vi "Lab Panel V5.29.vi"() -> ()   [LabVIEW 2013] (continued)
                            n2522 = Build Array(w4624) -> (w4612:dbl[])
                            n2523 = Build Array(w4625) -> (w4611:dbl[])
                            n2524 = Build Array(w4620) -> (w4616:dbl[])
                            n2525 = Build Array(w4618) -> (w4615:dbl[])
                            n2526 = Build Array(w4623) -> (w4610:dbl[])
                            n2527 = Build Array("AMPS ON", "AMPS OFF", "VOLTS", "PF", "TEMP Live", "TEMP Neut", "CYCLE") -> (w4593:string[])
                            n2528 = Bundle By Name("Y"=w4616, "t0"=w4609) -> (w4608:waveform(dbl))  [unwired: 1 in]
                            n2529 = Bundle By Name("Y"=w4615, "t0"=w4609) -> (w4607:waveform(dbl))  [unwired: 1 in]
                            n2530 = Bundle By Name("Y"=w4614, "t0"=w4609) -> (w4606:waveform(dbl))  [unwired: 1 in]
                            n2531 = Bundle By Name("Y"=w4613, "t0"=w4609) -> (w4605:waveform(dbl))  [unwired: 1 in]
                            n2532 = Bundle By Name("Y"=w4612, "t0"=w4609) -> (w4604:waveform(dbl))  [unwired: 1 in]
                            n2533 = Bundle By Name("Y"=w4611, "t0"=w4609) -> (w4603:waveform(dbl))  [unwired: 1 in]
                            n2534 = Bundle By Name("Y"=w4610, "t0"=w4609) -> (w4602:waveform(dbl))  [unwired: 1 in]
                            n2535 = Build Array(w4608, w4607, w4606, w4605, w4604, w4603, w4602) -> (w4601:waveform(dbl)[])
                            n2536 = TDMS Write(0:w4622, 5:"TEST VALUES", 7:w4593, 9:w4601) -> (4:w4592:refnum<k34>, 6:w4591:string, 15:w4590:errorcluster)  [unwired: 2 in, 1 out]
                            n2537 = TDMS Write(0:w4592, 5:w4591, 7:"TIME", 9:w4588, 11:w4590) -> (15:w4587:errorcluster)  [unwired: 1 in, 3 out]
                            n2538 = local write "data file error"(w4587) -> ()
                          }
                        }
                      }
                    }
                  }
                }
              }
              frame #8 {
                n2539 = case shown="True" w4626 {
                  tunnel: w4630 -> [_ w4635]
                  tunnel: w4629 -> [_ w4634]
                  tunnel: w4628 -> [_ w4632]
                  tunnel: w4627 -> [_ w4631]
                  frame False {
                  }
                  frame True {
                    n2540 = local read "DISP LAB05-1"() -> (w4636:T4)
                    n2541 = local read "SIG LAB05-1"() -> (w4637:T2)
                    n2542 = local read "ON L05-1"() -> (w4633:cluster{"amps":dbl, "volts":dbl, "pf":dbl})
                    n2543 = Unbundle(w4637) -> ("AMPS"=w4643:dbl, "VOLTS"=w4641:dbl, "PF"=w4640:dbl, "Tmp Live"=w4639:dbl, "Tmp Neut"=w4642:dbl)
                    n2544 = Unbundle(w4636) -> ("CYCLE"=w4638:dbl)  [unwired: 2 out]
                    n2545 = stacked-sequence {
                      tunnel: w4643 -> [w4647 w4666]
                      tunnel: w4642 -> [_ w4665]
                      tunnel: w4641 -> [w4646 w4664]
                      tunnel: w4640 -> [w4645 w4663]
                      tunnel: w4639 -> [_ w4662]
                      tunnel: w4638 -> [_ w4661]
                      tunnel: w4635 -> [_ w4660]
                      tunnel: w4634 -> [w4648 _]
                      tunnel: w4633 -> [w4644 w4658]
                      tunnel: w4632 -> [_ w4659]
                      tunnel: w4631 -> [_ w4654]
                      frame #0 {
                        n2546 = case shown="True" w4648 {
                          tunnel: w4647 -> [_ w4653]
                          tunnel: w4646 -> [_ w4652]
                          tunnel: w4645 -> [_ w4651]
                          tunnel: w4644 -> [_ w4649]
                          frame False {
                          }
                          frame True {
                            n2547 = Bundle(cluster=w4649, "amps"=w4653, "volts"=w4652, "pf"=w4651) -> (w4650:cluster{"amps":dbl, "volts":dbl, "pf":dbl})
                            n2548 = local write "ON L05-1"(w4650) -> ()
                          }
                        }
                      }
                      frame #1 {
                        n2549 = Unbundle(w4658) -> ("amps"=w4657:dbl, "volts"=w4656:dbl, "pf"=w4655:dbl)
                        n2550 = case shown="True" w4659 {
                          tunnel: w4666 -> [_ w4698]
                          tunnel: w4665 -> [_ w4705]
                          tunnel: w4664 -> [_ _]
                          tunnel: w4663 -> [_ _]
                          tunnel: w4662 -> [_ w4704]
                          tunnel: w4661 -> [_ w4703]
                          tunnel: w4660 -> [_ w4668]
                          tunnel: w4657 -> [_ w4700]
                          tunnel: w4656 -> [_ w4699]
                          tunnel: w4655 -> [_ w4697]
                          tunnel: w4654 -> [_ w4689]
                          frame False {
                          }
                          frame True {
                            n2551 = local read "TDMS LAB05-1"() -> (w4702:refnum<k34>)
                            n2552 = Build Array(w4699) -> (w4694:dbl[])
                            n2553 = Build Array(w4697) -> (w4693:dbl[])
                            n2554 = Build Array(w4704) -> (w4692:dbl[])
                            n2555 = Build Array(w4705) -> (w4691:dbl[])
                            n2556 = Build Array(w4700) -> (w4696:dbl[])
                            n2557 = Build Array(w4698) -> (w4695:dbl[])
                            n2558 = Build Array(w4703) -> (w4690:dbl[])
                            n2559 = Build Array("AMPS ON", "AMPS OFF", "VOLTS", "PF", "TEMP Live", "TEMP Neut", "CYCLE") -> (w4673:string[])
                            n2560 = Bundle By Name("Y"=w4696, "t0"=w4689) -> (w4688:waveform(dbl))  [unwired: 1 in]
                            n2561 = Bundle By Name("Y"=w4695, "t0"=w4689) -> (w4687:waveform(dbl))  [unwired: 1 in]
                            n2562 = Bundle By Name("Y"=w4694, "t0"=w4689) -> (w4686:waveform(dbl))  [unwired: 1 in]
                            n2563 = Bundle By Name("Y"=w4693, "t0"=w4689) -> (w4685:waveform(dbl))  [unwired: 1 in]
                            n2564 = Bundle By Name("Y"=w4692, "t0"=w4689) -> (w4684:waveform(dbl))  [unwired: 1 in]
                            n2565 = Bundle By Name("Y"=w4691, "t0"=w4689) -> (w4683:waveform(dbl))  [unwired: 1 in]
                            n2566 = Bundle By Name("Y"=w4690, "t0"=w4689) -> (w4682:waveform(dbl))  [unwired: 1 in]
                            n2567 = Build Array(w4688, w4687, w4686, w4685, w4684, w4683, w4682) -> (w4681:waveform(dbl)[])
                            n2568 = TDMS Write(0:w4702, 5:"TEST VALUES", 7:w4673, 9:w4681) -> (4:w4672:refnum<k34>, 6:w4671:string, 15:w4670:errorcluster)  [unwired: 2 in, 1 out]
                            n2569 = TDMS Write(0:w4672, 5:w4671, 7:"TIME", 9:w4668, 11:w4670) -> (15:w4667:errorcluster)  [unwired: 1 in, 3 out]
                            n2570 = local write "data file error"(w4667) -> ()
                          }
                        }
                      }
                    }
                  }
                }
              }
              frame #9 {
                n2571 = case shown="True" w4706 {
                  tunnel: w4710 -> [_ w4715]
                  tunnel: w4709 -> [_ w4714]
                  tunnel: w4708 -> [_ w4712]
                  tunnel: w4707 -> [_ w4711]
                  frame False {
                  }
                  frame True {
                    n2572 = local read "DISP LAB05-2"() -> (w4716:T4)
                    n2573 = local read "SIG LAB05-2"() -> (w4717:T2)
                    n2574 = local read "ON L05-2"() -> (w4713:cluster{"amps":dbl, "volts":dbl, "pf":dbl})
                    n2575 = Unbundle(w4717) -> ("AMPS"=w4723:dbl, "VOLTS"=w4721:dbl, "PF"=w4720:dbl, "Tmp Live"=w4719:dbl, "Tmp Neut"=w4722:dbl)
                    n2576 = Unbundle(w4716) -> ("CYCLE"=w4718:dbl)  [unwired: 2 out]
                    n2577 = stacked-sequence {
                      tunnel: w4723 -> [w4727 w4746]
                      tunnel: w4722 -> [_ w4745]
                      tunnel: w4721 -> [w4726 w4744]
                      tunnel: w4720 -> [w4725 w4743]
                      tunnel: w4719 -> [_ w4742]
                      tunnel: w4718 -> [_ w4741]
                      tunnel: w4715 -> [_ w4740]
                      tunnel: w4714 -> [w4728 _]
                      tunnel: w4713 -> [w4724 w4738]
                      tunnel: w4712 -> [_ w4739]
                      tunnel: w4711 -> [_ w4734]
                      frame #0 {
                        n2578 = case shown="True" w4728 {
                          tunnel: w4727 -> [_ w4733]
                          tunnel: w4726 -> [_ w4732]
                          tunnel: w4725 -> [_ w4731]
                          tunnel: w4724 -> [_ w4729]
                          frame False {
                          }
                          frame True {
                            n2579 = Bundle(cluster=w4729, "amps"=w4733, "volts"=w4732, "pf"=w4731) -> (w4730:cluster{"amps":dbl, "volts":dbl, "pf":dbl})
                            n2580 = local write "ON L05-2"(w4730) -> ()
                          }
                        }
                      }
                      frame #1 {
                        n2581 = Unbundle(w4738) -> ("amps"=w4737:dbl, "volts"=w4736:dbl, "pf"=w4735:dbl)
                        n2582 = case shown="True" w4739 {
                          tunnel: w4746 -> [_ w4778]
                          tunnel: w4745 -> [_ w4785]
                          tunnel: w4744 -> [_ _]
                          tunnel: w4743 -> [_ _]
                          tunnel: w4742 -> [_ w4784]
                          tunnel: w4741 -> [_ w4783]
                          tunnel: w4740 -> [_ w4748]
                          tunnel: w4737 -> [_ w4780]
                          tunnel: w4736 -> [_ w4779]
                          tunnel: w4735 -> [_ w4777]
                          tunnel: w4734 -> [_ w4769]
                          frame False {
                          }
                          frame True {
                            n2583 = local read "TDMS LAB05-2"() -> (w4782:refnum<k34>)
                            n2584 = Build Array(w4779) -> (w4774:dbl[])
                            n2585 = Build Array(w4777) -> (w4773:dbl[])
                            n2586 = Build Array(w4784) -> (w4772:dbl[])
                            n2587 = Build Array(w4785) -> (w4771:dbl[])
                            n2588 = Build Array(w4780) -> (w4776:dbl[])
                            n2589 = Build Array(w4778) -> (w4775:dbl[])
                            n2590 = Build Array(w4783) -> (w4770:dbl[])
                            n2591 = Build Array("AMPS ON", "AMPS OFF", "VOLTS", "PF", "TEMP Live", "TEMP Neut", "CYCLE") -> (w4753:string[])
                            n2592 = Bundle By Name("Y"=w4776, "t0"=w4769) -> (w4768:waveform(dbl))  [unwired: 1 in]
                            n2593 = Bundle By Name("Y"=w4775, "t0"=w4769) -> (w4767:waveform(dbl))  [unwired: 1 in]
                            n2594 = Bundle By Name("Y"=w4774, "t0"=w4769) -> (w4766:waveform(dbl))  [unwired: 1 in]
                            n2595 = Bundle By Name("Y"=w4773, "t0"=w4769) -> (w4765:waveform(dbl))  [unwired: 1 in]
                            n2596 = Bundle By Name("Y"=w4772, "t0"=w4769) -> (w4764:waveform(dbl))  [unwired: 1 in]
                            n2597 = Bundle By Name("Y"=w4771, "t0"=w4769) -> (w4763:waveform(dbl))  [unwired: 1 in]
                            n2598 = Bundle By Name("Y"=w4770, "t0"=w4769) -> (w4762:waveform(dbl))  [unwired: 1 in]
                            n2599 = Build Array(w4768, w4767, w4766, w4765, w4764, w4763, w4762) -> (w4761:waveform(dbl)[])
                            n2600 = TDMS Write(0:w4782, 5:"TEST VALUES", 7:w4753, 9:w4761) -> (4:w4752:refnum<k34>, 6:w4751:string, 15:w4750:errorcluster)  [unwired: 2 in, 1 out]
                            n2601 = TDMS Write(0:w4752, 5:w4751, 7:"TIME", 9:w4748, 11:w4750) -> (15:w4747:errorcluster)  [unwired: 1 in, 3 out]
                            n2602 = local write "data file error"(w4747) -> ()
                          }
                        }
                      }
                    }
                  }
                }
              }
            }
          }
          frame #15 {
            # "display test values on chart"
            n2603 = local read "jig cycle"() -> (w4790:dbl)
            n2604 = local read "on loops"() -> (w4792:dbl)
            n2605 = Add(x=w4792, y=4) -> (x+y=w4789:dbl)
            n2606 = Equal?(x=w4790, y=3) -> (x = y?=w4788:bool)
            n2607 = Equal?(x=w4790, y=w4789) -> (x = y?=w4787:bool)
            n2608 = Or(x=w4788, y=w4787) -> (x .or. y?=w4786:bool)
            "graph flag" <- w4786
            n2609 = global write "Global display 3.vi" "graph flag"(w4786) -> ()
            n2610 = case shown="True" w4786 {
              frame False {
              }
              frame True {
                n2611 = local read "SIG LAB05-1"() -> (w4835:T2)
                n2612 = local read "SIG LAB04-2"() -> (w4836:T2)
                n2613 = local read "SIG LAB05-2"() -> (w4834:T2)
                n2614 = local read "SIG LAB04-1"() -> (w4837:T2)
                n2615 = local read "SIG LAB03-1"() -> (w4839:T2)
                n2616 = local read "SIG LAB03-2"() -> (w4838:T2)
                n2617 = local read "SIG LAB01-1"() -> (w4843:T2)
                n2618 = local read "SIG LAB02-2"() -> (w4840:T2)
                n2619 = local read "SIG LAB02-1"() -> (w4841:T2)
                n2620 = local read "SIG LAB01-2"() -> (w4842:T2)
                n2621 = Unbundle(w4836) -> ("AMPS"=w4826:dbl, "VOLTS"=w4816:dbl, "Tmp Live"=w4806:dbl, "Tmp Neut"=w4796:dbl)  [unwired: 1 out]
                n2622 = Unbundle(w4835) -> ("AMPS"=w4825:dbl, "VOLTS"=w4815:dbl, "Tmp Live"=w4805:dbl, "Tmp Neut"=w4795:dbl)  [unwired: 1 out]
                n2623 = Unbundle(w4834) -> ("AMPS"=w4824:dbl, "VOLTS"=w4814:dbl, "Tmp Live"=w4804:dbl, "Tmp Neut"=w4794:dbl)  [unwired: 1 out]
                n2624 = Unbundle(w4837) -> ("AMPS"=w4827:dbl, "VOLTS"=w4817:dbl, "Tmp Live"=w4807:dbl, "Tmp Neut"=w4797:dbl)  [unwired: 1 out]
                n2625 = Unbundle(w4838) -> ("AMPS"=w4828:dbl, "VOLTS"=w4818:dbl, "Tmp Live"=w4808:dbl, "Tmp Neut"=w4798:dbl)  [unwired: 1 out]
                n2626 = Unbundle(w4839) -> ("AMPS"=w4829:dbl, "VOLTS"=w4819:dbl, "Tmp Live"=w4809:dbl, "Tmp Neut"=w4799:dbl)  [unwired: 1 out]
                n2627 = Unbundle(w4840) -> ("AMPS"=w4830:dbl, "VOLTS"=w4820:dbl, "Tmp Live"=w4810:dbl, "Tmp Neut"=w4800:dbl)  [unwired: 1 out]
                n2628 = Unbundle(w4841) -> ("AMPS"=w4831:dbl, "VOLTS"=w4821:dbl, "Tmp Live"=w4811:dbl, "Tmp Neut"=w4801:dbl)  [unwired: 1 out]
                n2629 = Unbundle(w4843) -> ("AMPS"=w4833:dbl, "VOLTS"=w4823:dbl, "Tmp Live"=w4813:dbl, "Tmp Neut"=w4803:dbl)  [unwired: 1 out]
                n2630 = Unbundle(w4842) -> ("AMPS"=w4832:dbl, "VOLTS"=w4822:dbl, "Tmp Live"=w4812:dbl, "Tmp Neut"=w4802:dbl)  [unwired: 1 out]
                n2631 = stacked-sequence {
                  tunnel: w4833 -> [w4875 _ _]
                  tunnel: w4832 -> [w4874 _ _]
                  tunnel: w4831 -> [w4865 _ _]
                  tunnel: w4830 -> [w4864 _ _]
                  tunnel: w4829 -> [w4854 _ _]
                  tunnel: w4828 -> [w4853 _ _]
                  tunnel: w4827 -> [_ w4898 _]
                  tunnel: w4826 -> [_ w4897 _]
                  tunnel: w4825 -> [_ w4887 _]
                  tunnel: w4824 -> [_ w4886 _]
                  tunnel: w4823 -> [w4872 _ _]
                  tunnel: w4822 -> [w4871 _ _]
                  tunnel: w4821 -> [w4862 _ _]
                  tunnel: w4820 -> [w4861 _ _]
                  tunnel: w4819 -> [w4852 _ _]
                  tunnel: w4818 -> [w4851 _ _]
                  tunnel: w4817 -> [_ w4896 _]
                  tunnel: w4816 -> [_ w4895 _]
                  tunnel: w4815 -> [_ w4885 _]
                  tunnel: w4814 -> [_ w4884 _]
                  tunnel: w4813 -> [w4869 _ _]
                  tunnel: w4812 -> [w4867 _ _]
                  tunnel: w4811 -> [w4858 _ _]
                  tunnel: w4810 -> [w4856 _ _]
                  tunnel: w4809 -> [w4850 _ _]
                  tunnel: w4808 -> [w4848 _ _]
                  tunnel: w4807 -> [_ w4894 _]
                  tunnel: w4806 -> [_ w4892 _]
                  tunnel: w4805 -> [_ w4883 _]
                  tunnel: w4804 -> [_ w4881 _]
                  tunnel: w4803 -> [w4868 _ _]
                  tunnel: w4802 -> [w4866 _ _]
                  tunnel: w4801 -> [w4857 _ _]
                  tunnel: w4800 -> [w4855 _ _]
                  tunnel: w4799 -> [w4849 _ _]
                  tunnel: w4798 -> [w4847 _ _]
                  tunnel: w4797 -> [_ w4893 _]
                  tunnel: w4796 -> [_ w4891 _]
                  tunnel: w4795 -> [_ w4882 _]
                  tunnel: w4794 -> [_ w4880 _]
                  frame #0 {
                    n2632 = Merge Signals(w4875, w4874) -> (→"LAB01 AMPS":dynamicdata)
                    n2633 = Merge Signals(w4872, w4871) -> (→"LAB01 VOLTS":dynamicdata)
                    n2634 = Merge Signals(w4852, w4851) -> (→"LAB03 VOLTS":dynamicdata)
                    n2635 = Merge Signals(w4869, w4868, w4867, w4866) -> (→"LAB01 deg C":dynamicdata)
                    n2636 = Merge Signals(w4865, w4864) -> (→"LAB02 AMPS":dynamicdata)
                    n2637 = Merge Signals(w4858, w4857, w4856, w4855) -> (→"LAB02 deg C":dynamicdata)
                    n2638 = Merge Signals(w4850, w4849, w4848, w4847) -> (→"LAB03 deg C":dynamicdata)
                    n2639 = Merge Signals(w4862, w4861) -> (→"LAB02 VOLTS":dynamicdata)
                    n2640 = Merge Signals(w4854, w4853) -> (→"LAB03 AMPS":dynamicdata)
                  }
                  frame #1 {
                    n2641 = Merge Signals(w4885, w4884) -> (→"LAB05 VOLTS":dynamicdata)
                    n2642 = Merge Signals(w4898, w4897) -> (→"LAB04 AMPS":dynamicdata)
                    n2643 = Merge Signals(w4887, w4886) -> (→"LAB05 AMPS":dynamicdata)
                    n2644 = Merge Signals(w4883, w4882, w4881, w4880) -> (→"LAB05 deg C":dynamicdata)
                    n2645 = Merge Signals(w4894, w4893, w4892, w4891) -> (→"LAB04 deg C":dynamicdata)
                    n2646 = Merge Signals(w4896, w4895) -> (→"LAB04 VOLTS":dynamicdata)
                  }
                  frame #2 {
                    n2647 = local read "LAB05 VOLTS"() -> (w4906:dynamicdata)
                    n2648 = local read "LAB04 VOLTS"() -> (w4907:dynamicdata)
                    n2649 = local read "LAB02 VOLTS"() -> (w4909:dynamicdata)
                    n2650 = local read "LAB03 VOLTS"() -> (w4908:dynamicdata)
                    n2651 = local read "LAB05 AMPS"() -> (w4912:dynamicdata)
                    n2652 = local read "LAB01 VOLTS"() -> (w4910:dynamicdata)
                    n2653 = local read "LAB04 AMPS"() -> (w4913:dynamicdata)
                    n2654 = local read "LAB03 AMPS"() -> (w4914:dynamicdata)
                    n2655 = local read "LAB03 deg C"() -> (w4902:dynamicdata)
                    n2656 = local read "LAB02 AMPS"() -> (w4915:dynamicdata)
                    n2657 = local read "LAB04 deg C"() -> (w4901:dynamicdata)
                    n2658 = local read "LAB05 deg C"() -> (w4900:dynamicdata)
                    n2659 = local read "LAB02 deg C"() -> (w4903:dynamicdata)
                    n2660 = local read "LAB01 deg C"() -> (w4904:dynamicdata)
                    n2661 = local read "LAB01 AMPS"() -> (w4916:dynamicdata)
                    n2662 = Merge Signals(w4904, w4903, w4902, w4901, w4900) -> (w4899:dynamicdata)
                    n2663 = Merge Signals(w4916, w4915, w4914, w4913, w4912) -> (w4911:dynamicdata)
                    n2664 = Merge Signals(w4910, w4909, w4908, w4907, w4906) -> (w4905:dynamicdata)
                    n2665 = global write "Global display 3.vi" "graph volts"(w4905) -> ()
                    n2666 = global write "Global display 3.vi" "graph deg C"(w4899) -> ()
                    n2667 = global write "Global display 3.vi" "graph amps"(w4911) -> ()
                  }
                }
              }
            }
          }
          frame #16 {
            # "check for amps fail"
            # "check for cycle test & temperature rise fail conditions"
            n2668 = local read "on loops"() -> (w4943:dbl)
            n2669 = local read "jig cycle"() -> (w4940:dbl)
            n2670 = local read "jig cycle"() -> (w4945:dbl)
            n2671 = Add(x=w4943, y=5.0) -> (x+y=w4941:dbl)
            n2672 = Equal?(x=w4940, y=w4941) -> (x = y?=w4936:bool)
            n2673 = local read "Fail Loops"() -> (w4917:dbl)
            n2674 = Equal?(x=w4945, y=3.0) -> (x = y?=w4938:bool)
            n2675 = global write "Global 1.vi" "fail count"(w4917) -> ()
            n2676 = stacked-sequence {
              tunnel: w4939 -> [w4948 _ _ _ _ _ _ _ _ _]
              tunnel: w4938 -> [w4949 w4969 w4989 w5009 w5029 w5049 w5069 w5089 w5109 w5129]
              tunnel: w4937 -> [w4946 _ _ _ _ _ _ _ _ _]
              tunnel: w4936 -> [w4947 w4968 w4988 w5008 w5028 w5048 w5068 w5088 w5108 w5128]
              tunnel: w4935 -> [_ w4967 _ _ _ _ _ _ _ _]
              tunnel: w4934 -> [_ w4966 _ _ _ _ _ _ _ _]
              tunnel: w4933 -> [_ _ w4987 _ _ _ _ _ _ _]
              tunnel: w4932 -> [_ _ w4986 _ _ _ _ _ _ _]
              tunnel: w4931 -> [_ _ _ w5007 _ _ _ _ _ _]
              tunnel: w4930 -> [_ _ _ w5006 _ _ _ _ _ _]
              tunnel: w4929 -> [_ _ _ _ w5027 _ _ _ _ _]
              tunnel: w4928 -> [_ _ _ _ w5026 _ _ _ _ _]
              tunnel: w4927 -> [_ _ _ _ _ w5047 _ _ _ _]
              tunnel: w4926 -> [_ _ _ _ _ w5046 _ _ _ _]
              tunnel: w4925 -> [_ _ _ _ _ _ w5067 _ _ _]
              tunnel: w4924 -> [_ _ _ _ _ _ w5066 _ _ _]
              tunnel: w4923 -> [_ _ _ _ _ _ _ w5087 _ _]
              tunnel: w4922 -> [_ _ _ _ _ _ _ w5086 _ _]
              tunnel: w4921 -> [_ _ _ _ _ _ _ _ w5107 _]
              tunnel: w4920 -> [_ _ _ _ _ _ _ _ w5106 _]
              tunnel: w4919 -> [_ _ _ _ _ _ _ _ _ w5127]
              tunnel: w4918 -> [_ _ _ _ _ _ _ _ _ w5126]
              frame #0 {
                # "LAB01-1"
                n2677 = case shown="True" w4946 {
                  tunnel: w4949 -> [_ w4962]
                  tunnel: w4948 -> [_ w4959]
                  tunnel: w4947 -> [_ w4958]
                  frame False {
                  }
                  frame True {
                    n2678 = local read "TEMP START LAB01-1"() -> (w4964:cluster{"TL":dbl, "TN":dbl})
                    n2679 = local read "RESULT LAB01-1"() -> (w4953:bool)
                    n2680 = local read "FAIL LAB01-1"() -> (w4956:cluster{"LO":dbl, "HI":dbl})
                    n2681 = local read "TDMS LAB01-1"() -> (w4963:refnum<k34>)
                    n2682 = local read "SET LAB01-1"() -> (w4960:T5)
                    n2683 = local read "DISP LAB01-1"() -> (w4961:T4)
                    n2684 = local read "SIG LAB01-1"() -> (w4965:T2)
                    n2685 = Bundle("FAIL LAB01-1"=w4956, "SIG LAB01-1"=w4965, "TEMP START LAB01-1"=w4964, "DISP LAB01-1"=w4961, "SET LAB01-1"=w4960, "TDMS LAB01-1"=w4963) -> (w4950:T33)  [unwired: 1 in]
                    n2686 = call "sub vi - cycle&temp fail v7.vi"("Amps Lo?"=w4962, "Input Cluster"=w4950, "SELECT"=w4959, "Amps Hi?"=w4958, "Result In"=w4953) -> ("(FAIL) out"=w4955:cluster{"FAIL LO":dbl, "FAIL HI":dbl}, "(DISP) out"=w4951:T4, "T-RISE"=w4952:cluster{"T-RISE (L)":dbl, "T-RISE (N)":dbl}, "Result Out"=w4954:bool, "file error"=w4957:errorcluster)  [unwired: 10 in]
                    n2687 = local write "TEMP RISE LAB01-1"(w4952) -> ()
                    n2688 = local write "FAIL LAB01-1"(w4955) -> ()
                    n2689 = local write "DISP LAB01-1"(w4951) -> ()
                    n2690 = local write "RESULT LAB01-1"(w4954) -> ()
                    n2691 = local write "data file error"(w4957) -> ()
                  }
                }
              }
              frame #1 {
                # "LAB01-2"
                n2692 = case shown="True" w4967 {
                  tunnel: w4969 -> [_ w4982]
                  tunnel: w4966 -> [_ w4979]
                  tunnel: w4968 -> [_ w4978]
                  frame False {
                  }
                  frame True {
                    n2693 = local read "TEMP START LAB01-2"() -> (w4984:cluster{"TL":dbl, "TN":dbl})
                    n2694 = local read "FAIL LAB01-2"() -> (w4975:cluster{"LO":dbl, "HI":dbl})
                    n2695 = local read "TDMS LAB01-2"() -> (w4983:refnum<k34>)
                    n2696 = local read "SET LAB01-2"() -> (w4980:T5)
                    n2697 = local read "DISP LAB01-2"() -> (w4981:T4)
                    n2698 = local read "RESULT LAB01-2"() -> (w4972:bool)
                    n2699 = local read "SIG LAB01-2"() -> (w4985:T2)
                    n2700 = Bundle("FAIL LAB01-2"=w4975, "SIG LAB01-2"=w4985, "TEMP START LAB01-2"=w4984, "DISP LAB01-2"=w4981, "SET LAB01-2"=w4980, "TDMS LAB01-2"=w4983) -> (w4970:T34)  [unwired: 1 in]
                    n2701 = call "sub vi - cycle&temp fail v7.vi"("Amps Lo?"=w4982, "Input Cluster"=w4970, "SELECT"=w4979, "Amps Hi?"=w4978, "Result In"=w4972) -> ("(FAIL) out"=w4974:cluster{"FAIL LO":dbl, "FAIL HI":dbl}, "(DISP) out"=w4977:T4, "T-RISE"=w4971:cluster{"T-RISE (L)":dbl, "T-RISE (N)":dbl}, "Result Out"=w4973:bool, "file error"=w4976:errorcluster)  [unwired: 10 in]
                    n2702 = local write "TEMP RISE LAB01-2"(w4971) -> ()
                    n2703 = local write "FAIL LAB01-2"(w4974) -> ()
                    n2704 = local write "DISP LAB01-2"(w4977) -> ()
                    n2705 = local write "RESULT LAB01-2"(w4973) -> ()
                    n2706 = local write "data file error"(w4976) -> ()
                  }
                }
              }
              frame #2 {
                # "LAB02-1"
                n2707 = case shown="True" w4987 {
                  tunnel: w4989 -> [_ w5002]
                  tunnel: w4986 -> [_ w4999]
                  tunnel: w4988 -> [_ w4998]
                  frame False {
                  }
                  frame True {
                    n2708 = local read "TEMP START LAB02-1"() -> (w5004:cluster{"TL":dbl, "TN":dbl})
                    n2709 = local read "FAIL LAB02-1"() -> (w4995:cluster{"LO":dbl, "HI":dbl})
                    n2710 = local read "TDMS LAB02-1"() -> (w5003:refnum<k34>)
                    n2711 = local read "SET LAB02-1"() -> (w5000:T5)
                    n2712 = local read "DISP LAB02-1"() -> (w5001:T4)
                    n2713 = local read "SIG LAB02-1"() -> (w5005:T2)
                    n2714 = local read "RESULT LAB02-1"() -> (w4992:bool)
                    n2715 = Bundle("FAIL LAB02-1"=w4995, "SIG LAB02-1"=w5005, "TEMP START LAB02-1"=w5004, "DISP LAB02-1"=w5001, "SET LAB02-1"=w5000, "TDMS LAB02-1"=w5003) -> (w4990:T35)  [unwired: 1 in]
                    n2716 = call "sub vi - cycle&temp fail v7.vi"("Amps Lo?"=w5002, "Input Cluster"=w4990, "SELECT"=w4999, "Amps Hi?"=w4998, "Result In"=w4992) -> ("(FAIL) out"=w4994:cluster{"FAIL LO":dbl, "FAIL HI":dbl}, "(DISP) out"=w4997:T4, "T-RISE"=w4991:cluster{"T-RISE (L)":dbl, "T-RISE (N)":dbl}, "Result Out"=w4993:bool, "file error"=w4996:errorcluster)  [unwired: 10 in]
                    n2717 = local write "TEMP RISE LAB02-1"(w4991) -> ()
                    n2718 = local write "FAIL LAB02-1"(w4994) -> ()
                    n2719 = local write "DISP LAB02-1"(w4997) -> ()
                    n2720 = local write "RESULT LAB02-1"(w4993) -> ()
                    n2721 = local write "data file error"(w4996) -> ()
                  }
                }
              }
              frame #3 {
                # "LAB02-2"
                n2722 = case shown="True" w5007 {
                  tunnel: w5009 -> [_ w5022]
                  tunnel: w5006 -> [_ w5019]
                  tunnel: w5008 -> [_ w5018]
                  frame False {
                  }
                  frame True {
                    n2723 = local read "TEMP START LAB02-2"() -> (w5024:cluster{"TL":dbl, "TN":dbl})
                    n2724 = local read "FAIL LAB02-2"() -> (w5015:cluster{"LO":dbl, "HI":dbl})
                    n2725 = local read "TDMS LAB02-2"() -> (w5023:refnum<k34>)
                    n2726 = local read "SET LAB02-2"() -> (w5020:T5)
                    n2727 = local read "DISP LAB02-2"() -> (w5021:T4)
                    n2728 = local read "SIG LAB02-2"() -> (w5025:T2)
                    n2729 = local read "RESULT LAB02-2"() -> (w5012:bool)
                    n2730 = Bundle("FAIL LAB02-2"=w5015, "SIG LAB02-2"=w5025, "TEMP START LAB02-2"=w5024, "DISP LAB02-2"=w5021, "SET LAB02-2"=w5020, "TDMS LAB02-2"=w5023) -> (w5010:T36)  [unwired: 1 in]
                    n2731 = call "sub vi - cycle&temp fail v7.vi"("Amps Lo?"=w5022, "Input Cluster"=w5010, "SELECT"=w5019, "Amps Hi?"=w5018, "Result In"=w5012) -> ("(FAIL) out"=w5014:cluster{"FAIL LO":dbl, "FAIL HI":dbl}, "(DISP) out"=w5017:T4, "T-RISE"=w5011:cluster{"T-RISE (L)":dbl, "T-RISE (N)":dbl}, "Result Out"=w5013:bool, "file error"=w5016:errorcluster)  [unwired: 10 in]
                    n2732 = local write "TEMP RISE LAB02-2"(w5011) -> ()
                    n2733 = local write "FAIL LAB02-2"(w5014) -> ()
                    n2734 = local write "DISP LAB02-2"(w5017) -> ()
                    n2735 = local write "RESULT LAB02-2"(w5013) -> ()
                    n2736 = local write "data file error"(w5016) -> ()
                  }
                }
              }
              frame #4 {
                # "LAB03-1"
                n2737 = case shown="True" w5027 {
                  tunnel: w5029 -> [_ w5042]
                  tunnel: w5026 -> [_ w5039]
                  tunnel: w5028 -> [_ w5038]
                  frame False {
                  }
                  frame True {
                    n2738 = local read "TEMP START LAB03-1"() -> (w5044:cluster{"TL":dbl, "TN":dbl})
                    n2739 = local read "FAIL LAB03-1"() -> (w5035:cluster{"LO":dbl, "HI":dbl})
                    n2740 = local read "TDMS LAB03-1"() -> (w5043:refnum<k34>)
                    n2741 = local read "SET LAB03-1"() -> (w5040:T5)
                    n2742 = local read "DISP LAB03-1"() -> (w5041:T4)
                    n2743 = local read "SIG LAB03-1"() -> (w5045:T2)
                    n2744 = local read "RESULT LAB03-1"() -> (w5032:bool)
                    n2745 = Bundle("FAIL LAB03-1"=w5035, "SIG LAB03-1"=w5045, "TEMP START LAB03-1"=w5044, "DISP LAB03-1"=w5041, "SET LAB03-1"=w5040, "TDMS LAB03-1"=w5043) -> (w5030:T37)  [unwired: 1 in]
                    n2746 = call "sub vi - cycle&temp fail v7.vi"("Amps Lo?"=w5042, "Input Cluster"=w5030, "SELECT"=w5039, "Amps Hi?"=w5038, "Result In"=w5032) -> ("(FAIL) out"=w5034:cluster{"FAIL LO":dbl, "FAIL HI":dbl}, "(DISP) out"=w5037:T4, "T-RISE"=w5031:cluster{"T-RISE (L)":dbl, "T-RISE (N)":dbl}, "Result Out"=w5033:bool, "file error"=w5036:errorcluster)  [unwired: 10 in]
                    n2747 = local write "TEMP RISE LAB03-1"(w5031) -> ()
                    n2748 = local write "FAIL LAB03-1"(w5034) -> ()
                    n2749 = local write "DISP LAB03-1"(w5037) -> ()
                    n2750 = local write "RESULT LAB03-1"(w5033) -> ()
                    n2751 = local write "data file error"(w5036) -> ()
                  }
                }
              }
              frame #5 {
                # "LAB03-2"
                n2752 = case shown="True" w5047 {
                  tunnel: w5049 -> [_ w5062]
                  tunnel: w5046 -> [_ w5059]
                  tunnel: w5048 -> [_ w5058]
                  frame False {
                  }
                  frame True {
                    n2753 = local read "TEMP START LAB03-2"() -> (w5064:cluster{"TL":dbl, "TN":dbl})
                    n2754 = local read "FAIL LAB03-2"() -> (w5055:cluster{"LO":dbl, "HI":dbl})
                    n2755 = local read "TDMS LAB03-2"() -> (w5063:refnum<k34>)
                    n2756 = local read "SET LAB03-2"() -> (w5060:T5)
                    n2757 = local read "DISP LAB03-2"() -> (w5061:T4)
                    n2758 = local read "RESULT LAB03-2"() -> (w5052:bool)
                    n2759 = local read "SIG LAB03-2"() -> (w5065:T2)
                    n2760 = Bundle("FAIL LAB03-2"=w5055, "SIG LAB03-2"=w5065, "TEMP START LAB03-2"=w5064, "DISP LAB03-2"=w5061, "SET LAB03-2"=w5060, "TDMS LAB03-2"=w5063) -> (w5050:T38)  [unwired: 1 in]
                    n2761 = call "sub vi - cycle&temp fail v7.vi"("Amps Lo?"=w5062, "Input Cluster"=w5050, "SELECT"=w5059, "Amps Hi?"=w5058, "Result In"=w5052) -> ("(FAIL) out"=w5054:cluster{"FAIL LO":dbl, "FAIL HI":dbl}, "(DISP) out"=w5057:T4, "T-RISE"=w5051:cluster{"T-RISE (L)":dbl, "T-RISE (N)":dbl}, "Result Out"=w5053:bool, "file error"=w5056:errorcluster)  [unwired: 10 in]
                    n2762 = local write "FAIL LAB03-2"(w5054) -> ()
                    n2763 = local write "TEMP RISE LAB03-2"(w5051) -> ()
                    n2764 = local write "DISP LAB03-2"(w5057) -> ()
                    n2765 = local write "RESULT LAB03-2"(w5053) -> ()
                    n2766 = local write "data file error"(w5056) -> ()
                  }
                }
              }
              frame #6 {
                # "LAB04-1"
                n2767 = case shown="True" w5067 {
                  tunnel: w5069 -> [_ w5082]
                  tunnel: w5066 -> [_ w5079]
                  tunnel: w5068 -> [_ w5078]
                  frame False {
                  }
                  frame True {
                    n2768 = local read "TEMP START LAB04-1"() -> (w5084:cluster{"TL":dbl, "TN":dbl})
                    n2769 = local read "FAIL LAB04-1"() -> (w5075:cluster{"LO":dbl, "HI":dbl})
                    n2770 = local read "TDMS LAB04-1"() -> (w5083:refnum<k34>)
                    n2771 = local read "SET LAB04-1"() -> (w5080:T5)
                    n2772 = local read "DISP LAB04-1"() -> (w5081:T4)
                    n2773 = local read "SIG LAB04-1"() -> (w5085:T2)
                    n2774 = local read "RESULT LAB04-1"() -> (w5072:bool)
                    n2775 = Bundle("FAIL LAB04-1"=w5075, "SIG LAB04-1"=w5085, "TEMP START LAB04-1"=w5084, "DISP LAB04-1"=w5081, "SET LAB04-1"=w5080, "TDMS LAB04-1"=w5083) -> (w5070:T39)  [unwired: 1 in]
                    n2776 = call "sub vi - cycle&temp fail v7.vi"("Amps Lo?"=w5082, "Input Cluster"=w5070, "SELECT"=w5079, "Amps Hi?"=w5078, "Result In"=w5072) -> ("(FAIL) out"=w5074:cluster{"FAIL LO":dbl, "FAIL HI":dbl}, "(DISP) out"=w5077:T4, "T-RISE"=w5071:cluster{"T-RISE (L)":dbl, "T-RISE (N)":dbl}, "Result Out"=w5073:bool, "file error"=w5076:errorcluster)  [unwired: 10 in]
                    n2777 = local write "TEMP RISE LAB04-1"(w5071) -> ()
                    n2778 = local write "FAIL LAB04-1"(w5074) -> ()
                    n2779 = local write "DISP LAB04-1"(w5077) -> ()
                    n2780 = local write "RESULT LAB04-1"(w5073) -> ()
                    n2781 = local write "data file error"(w5076) -> ()
                  }
                }
              }
              frame #7 {
                # "LAB04-2"
                n2782 = case shown="True" w5087 {
                  tunnel: w5089 -> [_ w5102]
                  tunnel: w5086 -> [_ w5099]
                  tunnel: w5088 -> [_ w5098]
                  frame False {
                  }
                  frame True {
                    n2783 = local read "TEMP START LAB04-2"() -> (w5104:cluster{"TL":dbl, "TN":dbl})
                    n2784 = local read "FAIL LAB04-2"() -> (w5095:cluster{"LO":dbl, "HI":dbl})
                    n2785 = local read "TDMS LAB04-2"() -> (w5103:refnum<k34>)
                    n2786 = local read "SET LAB04-2"() -> (w5100:T5)
                    n2787 = local read "DISP LAB04-2"() -> (w5101:T4)
                    n2788 = local read "SIG LAB04-2"() -> (w5105:T2)
                    n2789 = local read "RESULT LAB04-2"() -> (w5092:bool)
                    n2790 = Bundle("FAIL LAB04-2"=w5095, "SIG LAB04-2"=w5105, "TEMP START LAB04-2"=w5104, "DISP LAB04-2"=w5101, "SET LAB04-2"=w5100, "TDMS LAB04-2"=w5103) -> (w5090:T40)  [unwired: 1 in]
                    n2791 = call "sub vi - cycle&temp fail v7.vi"("Amps Lo?"=w5102, "Input Cluster"=w5090, "SELECT"=w5099, "Amps Hi?"=w5098, "Result In"=w5092) -> ("(FAIL) out"=w5094:cluster{"FAIL LO":dbl, "FAIL HI":dbl}, "(DISP) out"=w5097:T4, "T-RISE"=w5091:cluster{"T-RISE (L)":dbl, "T-RISE (N)":dbl}, "Result Out"=w5093:bool, "file error"=w5096:errorcluster)  [unwired: 10 in]
                    n2792 = local write "TEMP RISE LAB04-2"(w5091) -> ()
                    n2793 = local write "FAIL LAB04-2"(w5094) -> ()
                    n2794 = local write "DISP LAB04-2"(w5097) -> ()
                    n2795 = local write "RESULT LAB04-2"(w5093) -> ()
                    n2796 = local write "data file error"(w5096) -> ()
                  }
                }
              }
              frame #8 {
                # "LAB05-1"
                n2797 = case shown="True" w5107 {
                  tunnel: w5109 -> [_ w5122]
                  tunnel: w5106 -> [_ w5119]
                  tunnel: w5108 -> [_ w5118]
                  frame False {
                  }
                  frame True {
                    n2798 = local read "TEMP START LAB05-1"() -> (w5124:cluster{"TL":dbl, "TN":dbl})
                    n2799 = local read "FAIL LAB05-1"() -> (w5115:cluster{"LO":dbl, "HI":dbl})
                    n2800 = local read "TDMS LAB05-1"() -> (w5123:refnum<k34>)
                    n2801 = local read "SET LAB05-1"() -> (w5120:T5)
                    n2802 = local read "DISP LAB05-1"() -> (w5121:T4)
                    n2803 = local read "SIG LAB05-1"() -> (w5125:T2)
                    n2804 = local read "RESULT LAB05-1"() -> (w5112:bool)
                    n2805 = Bundle("FAIL LAB05-1"=w5115, "SIG LAB05-1"=w5125, "TEMP START LAB05-1"=w5124, "DISP LAB05-1"=w5121, "SET LAB05-1"=w5120, "TDMS LAB05-1"=w5123) -> (w5110:T41)  [unwired: 1 in]
                    n2806 = call "sub vi - cycle&temp fail v7.vi"("Amps Lo?"=w5122, "Input Cluster"=w5110, "SELECT"=w5119, "Amps Hi?"=w5118, "Result In"=w5112) -> ("(FAIL) out"=w5114:cluster{"FAIL LO":dbl, "FAIL HI":dbl}, "(DISP) out"=w5117:T4, "T-RISE"=w5111:cluster{"T-RISE (L)":dbl, "T-RISE (N)":dbl}, "Result Out"=w5113:bool, "file error"=w5116:errorcluster)  [unwired: 10 in]
                    n2807 = local write "TEMP RISE LAB05-1"(w5111) -> ()
                    n2808 = local write "FAIL LAB05-1"(w5114) -> ()
                    n2809 = local write "DISP LAB05-1"(w5117) -> ()
                    n2810 = local write "RESULT LAB05-1"(w5113) -> ()
                    n2811 = local write "data file error"(w5116) -> ()
                  }
                }
              }
              frame #9 {
                # "LAB05-2"
                n2812 = case shown="True" w5127 {
                  tunnel: w5129 -> [_ w5142]
                  tunnel: w5126 -> [_ w5139]
                  tunnel: w5128 -> [_ w5138]
                  frame False {
                  }
                  frame True {
                    n2813 = local read "TEMP START LAB05-2"() -> (w5144:cluster{"TL":dbl, "TN":dbl})
                    n2814 = local read "FAIL LAB05-2"() -> (w5135:cluster{"LO":dbl, "HI":dbl})
                    n2815 = local read "TDMS LAB05-2"() -> (w5143:refnum<k34>)
                    n2816 = local read "SET LAB05-2"() -> (w5140:T5)
                    n2817 = local read "DISP LAB05-2"() -> (w5141:T4)
                    n2818 = local read "SIG LAB05-2"() -> (w5145:T2)
                    n2819 = local read "RESULT LAB05-2"() -> (w5132:bool)
                    n2820 = Bundle("FAIL LAB05-2"=w5135, "SIG LAB05-2"=w5145, "TEMP START LAB05-2"=w5144, "DISP LAB05-2"=w5141, "SET LAB05-2"=w5140, "TDMS LAB05-2"=w5143) -> (w5130:T42)  [unwired: 1 in]
                    n2821 = call "sub vi - cycle&temp fail v7.vi"("Amps Lo?"=w5142, "Input Cluster"=w5130, "SELECT"=w5139, "Amps Hi?"=w5138, "Result In"=w5132) -> ("(FAIL) out"=w5134:cluster{"FAIL LO":dbl, "FAIL HI":dbl}, "(DISP) out"=w5137:T4, "T-RISE"=w5131:cluster{"T-RISE (L)":dbl, "T-RISE (N)":dbl}, "Result Out"=w5133:bool, "file error"=w5136:errorcluster)  [unwired: 10 in]
                    n2822 = local write "TEMP RISE LAB05-2"(w5131) -> ()
                    n2823 = local write "FAIL LAB05-2"(w5134) -> ()
                    n2824 = local write "DISP LAB05-2"(w5137) -> ()
                    n2825 = local write "RESULT LAB05-2"(w5133) -> ()
                    n2826 = local write "data file error"(w5136) -> ()
                  }
                }
              }
            }
          }
          frame #17 {
            # "run calibration routine"
            n2827 = local read "SET (cal)"() -> (w5146:bool)
            n2828 = case shown="True" w5146 {
              frame False {
              }
              frame True {
                n2829 = stacked-sequence {
                  seq-local: [w5147 _ _] -> [_ w5149 _]
                  frame #0 {
                    n2830 = call "CALIBRATION PASSWORD"() -> ("PASSWORD"=w5147:string)  [unwired: 17 in, 2 out]
                  }
                  frame #1 {
                    n2831 = Equal?(x=w5149, y="7777") -> (x = y?=w5148:bool)
                    n2832 = case shown="True" w5148 {
                      frame False {
                      }
                      frame True {
                        n2833 = stacked-sequence {
                          frame #0 {
                            n2834 = local read "SAMPLES"() -> (w5151:dbl)
                            n2835 = local read "AI Task2"() -> (w5152:dbl)
                            n2836 = local read "AI Task1"() -> (w5153:dbl)
                            n2837 = local read "AI Task0"() -> (w5154:dbl)
                            n2838 = local read "Temp Test Cal"() -> (w5155:dbl)
                            n2839 = call "sub vi - calibration v2.vi"("Samples"=w5151, "Task2"=w5152, "Task1"=w5153, "Task0"=w5154, "Temp Test Cal"=w5155) -> ()  [unwired: 7 in]
                          }
                          frame #1 {
                            n2840 = call "sub vi - get calibration values v1.vi"() -> ("TEMP REF CAL"=w5156:dbl, "LAB01 (CAL)"=w5161:T14, "LAB02 (CAL)"=w5160:T15, "LAB03 (CAL)"=w5159:T14, "LAB04 (CAL)"=w5158:T14, "calibration file error out"=w5162:errorcluster, "LAB05 (CAL)"=w5157:T14)  [unwired: 9 in]
                            n2841 = local write "TEMP REF cal"(w5156) -> ()
                            n2842 = local write "cal file error out"(w5162) -> ()
                            n2843 = local write "CAL LAB04"(w5158) -> ()
                            n2844 = local write "CAL LAB05"(w5157) -> ()
                            n2845 = local write "CAL LAB01"(w5161) -> ()
                            n2846 = local write "CAL LAB02"(w5160) -> ()
                            n2847 = local write "CAL LAB03"(w5159) -> ()
                          }
                        }
                      }
                    }
                  }
                  frame #2 {
                    n2848 = local write "SET (cal)"(FALSE) -> ()
                  }
                }
              }
            }
          }
          frame #18 {
            # "save certain settings to file"
            n2849 = String To Path(string="c:\\crabtree\\Set Up\\") -> (path=w5165:path)
            n2850 = Build Path(base path=w5165, name or relative path="settings.bin") -> (appended path=w5167:path)
            n2851 = Build Path(base path=w5165, name or relative path="mail.bin") -> (appended path=w5164:path)
            n2852 = Create Folder(path (use dialog)=w5165) -> (error out=w5170:errorcluster)  [unwired: 2 in, 2 out]
            n2853 = call <vilib>:"Clear Errors.vi"("error in (no error)"=w5170) -> ()  [unwired: 6 in, 1 out]
            n2854 = stacked-sequence {
              seq-local: [w5182 _] -> [_ w5195]
              tunnel: w5167 -> [_ w5196]
              tunnel: w5164 -> [_ w5194]
              frame #0 {
                n2855 = local read "C drive data root dir"() -> (w5181:path)
                n2856 = local read "Select COM port"() -> (w5178:refnum<visa-resource-name>)
                n2857 = local read "Network Directory"() -> (w5187:path)
                n2858 = local read "SET LAB05-2"() -> (w5186:T5)
                n2859 = local read "SET LAB05-1"() -> (w5185:T5)
                n2860 = local read "SET LAB04-2"() -> (w5184:T5)
                n2861 = local read "SET LAB03-2"() -> (w5188:T5)
                n2862 = local read "SET LAB04-1"() -> (w5183:T5)
                n2863 = local read "SET LAB03-1"() -> (w5189:T5)
                n2864 = local read "SET LAB02-2"() -> (w5190:T5)
                n2865 = local read "SET LAB02-1"() -> (w5191:T5)
                n2866 = local read "Temp Delay Lps"() -> (w5177:dbl)
                n2867 = local read "Amps Fail level"() -> (w5173:dbl)
                n2868 = local read "SET LAB01-2"() -> (w5192:T5)
                n2869 = local read "Temp Test Cal"() -> (w5174:dbl)
                n2870 = local read "SET LAB01-1"() -> (w5193:T5)
                n2871 = local read "Mail Test File To:"() -> (w5172:string)
                n2872 = local read "Temp Value"() -> (w5176:dbl)
                n2873 = local read "Fail Loops"() -> (w5175:dbl)
                n2874 = local read "Mail Test Fail"() -> (w5171:bool)
                n2875 = local read "RATE (Hz)"() -> (w5180:dbl)
                n2876 = local read "SAMPLES"() -> (w5179:dbl)
                n2877 = Bundle("SET LAB01-1"=w5193, "SET LAB01-2"=w5192, "SET LAB02-1"=w5191, "SET LAB02-2"=w5190, "SET LAB03-1"=w5189, "SET LAB03-2"=w5188, "SET LAB04-1"=w5183, "SET LAB04-2"=w5184, "SET LAB05-1"=w5185, "SET LAB05-2"=w5186, "Network Directory"=w5187, "C drive data root dir"=w5181, "RATE (Hz)"=w5180, "SAMPLES"=w5179, "Select COM port"=w5178, "Temp Delay Lps"=w5177, "Temp Value"=w5176, "Fail Loops"=w5175, "Temp Test Cal"=w5174, "Amps Fail level"=w5173, "Mail Test File To:"=w5172, "Mail Test Fail"=w5171) -> (w5182:T22)  [unwired: 1 in]
              }
              frame #1 {
                n2878 = event shown="[1] \"SET LAB01-1\", \"SET LAB01-2\", \"SET LAB02-1\", \"SET LAB02-2\", \"SET LAB03-1\", \"SET LAB03-2\", \"SET LAB04-1\", \"SET LAB04-2\", \"SET LAB05-1\", \"SET LAB05-2\", \"Network Directory\", \"C drive data root dir\", \"RATE (Hz)\", \"SAMPLES\", \"Select COM port\", \"Temp Delay Lps\", \"Temp Value\", \"Fail Loops\", \"Temp Test Cal\", \"Amps Fail level\", \"Mail Test File To:\", \"Mail Test Fail\": Value Change" {
                  selector: _ -> [_ _ _]
                  dyn-events: _ -> [_ _ _]
                  timeout: 10.0 -> [_ _ _]
                  tunnel: w5196 -> [_ w5198 _]
                  tunnel: w5195 -> [_ w5199 _]
                  tunnel: w5194 -> [_ _ w5210]
                  event Timeout {
                    n2879 = event-data() -> ()  [unwired: 1 in, 3 out]
                  }
                  event "SET LAB01-1", "SET LAB01-2", "SET LAB02-1", "SET LAB02-2", "SET LAB03-1", "SET LAB03-2", "SET LAB04-1", "SET LAB04-2", "SET LAB05-1", "SET LAB05-2", "Network Directory", "C drive data root dir", "RATE (Hz)", "SAMPLES", "Select COM port", "Temp Delay Lps", "Temp Value", "Fail Loops", "Temp Test Cal", "Amps Fail level", "Mail Test File To:", "Mail Test Fail": Value Change {
                    n2880 = event-data() -> ()  [unwired: 1 in, 6 out]
                    n2881 = Open/Create/Replace File(file path (use dialog)=w5198, operation (0:open)=T17."replace or create") -> (refnum out=w5204:refnum<file>, error out=w5203:errorcluster)  [unwired: 4 in, 1 out]
                    n2882 = Write to Binary File(file (use dialog)=w5204, data=w5199, error in=w5203) -> (refnum out=w5202:refnum<file>, error out=w5201:errorcluster)  [unwired: 3 in, 1 out]
                    n2883 = Close File(refnum=w5202, error in=w5201) -> (error out=w5200:errorcluster)  [unwired: 1 out]
                    n2884 = local write "data file error"(w5200) -> ()
                  }
                  event "MAIL SETTINGS.OUT SERVER ADDRESS", "MAIL SETTINGS.FROM ACCOUNT", "MAIL SETTINGS.USER NAME", "MAIL SETTINGS.PASSWORD", "Auto Mail Send", "TO (string):": Value Change {
                    n2885 = event-data() -> ()  [unwired: 1 in, 6 out]
                    n2886 = local read "MAIL SETTINGS"() -> (w5209:T7)
                    n2887 = local read "Auto Mail Send"() -> (w5207:bool)
                    n2888 = local read "TO (string):"() -> (w5206:string)
                    n2889 = Open/Create/Replace File(file path (use dialog)=w5210, operation (0:open)=T17."replace or create") -> (refnum out=w5215:refnum<file>, error out=w5214:errorcluster)  [unwired: 4 in, 1 out]
                    n2890 = Bundle("MAIL SETTINGS"=w5209, "Auto Mail Send"=w5207, "TO (string):"=w5206) -> (w5208:T43)  [unwired: 1 in]
                    n2891 = Write to Binary File(file (use dialog)=w5215, data=w5208, error in=w5214) -> (refnum out=w5213:refnum<file>, error out=w5212:errorcluster)  [unwired: 3 in, 1 out]
                    n2892 = Close File(refnum=w5213, error in=w5212) -> (error out=w5211:errorcluster)  [unwired: 1 out]
                    n2893 = local write "data file error"(w5211) -> ()
                  }
                }
              }
            }
          }
          frame #19 {
            # "mail control"
            n2894 = local read "MAIL SETTINGS"() -> (w5232:T7)
            n2895 = local read "Auto Mail Send"() -> (w5218:bool)
